vi "Fe Material Properties.vi"(6 "m-nm Fe":dbl, 9 "Fe Thickness":dbl, 10 "Energy (Heat; I^2R)":dbl, 11 "NS Base Area":dbl) -> (1 "Mass Fe":dbl, 2 "Delta Temp Change Fe":dbl, 3 "Fe Specfic Heat Capacity":dbl, 4 "Fe Density":dbl, 5 "Fe Thickness 2":dbl, 7 "Volume Fe":dbl, 8 "mc":dbl)   [LabVIEW 2020]
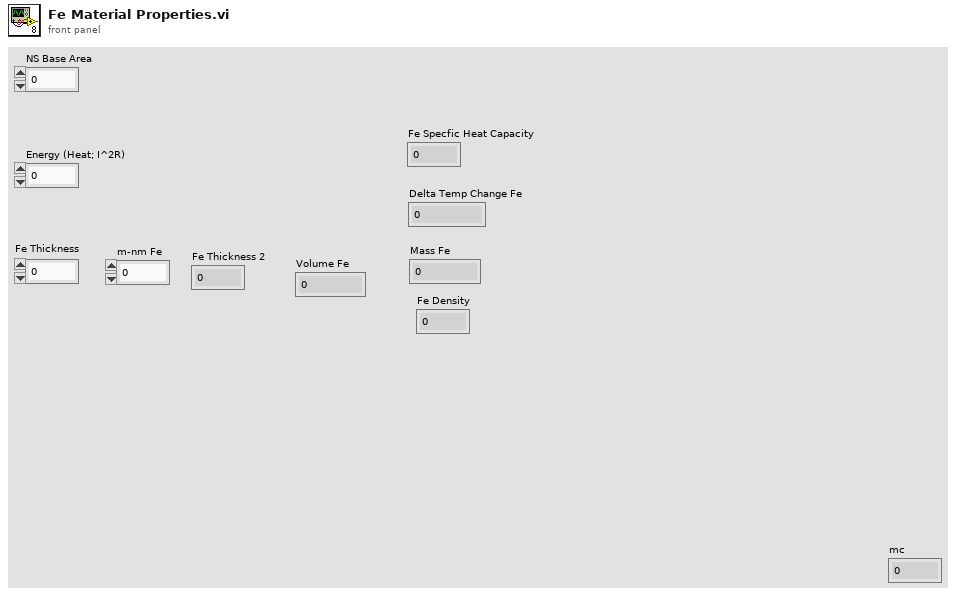
[diagram p1: front panel]
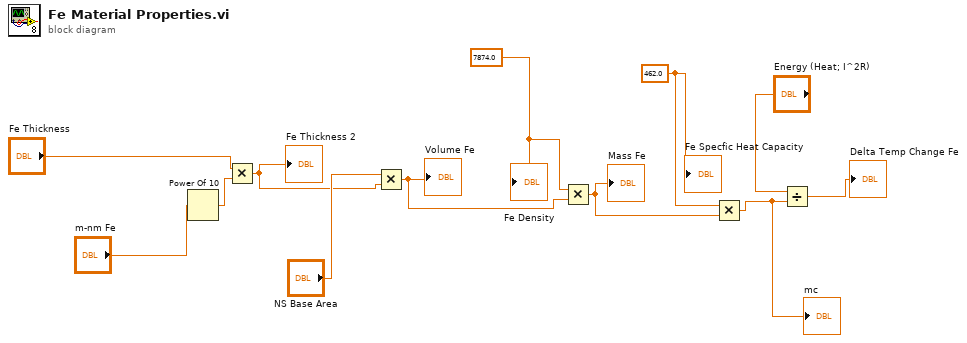
[diagram p0: block diagram]
diagram:
  w12 = 462.0 ("Silicon Specfic Heat Capacity 6")
  w6 = 7874.0 ("Silicon Density 6")
  n1 = Power Of 10(x="m-nm Fe") -> (10^x=w2:dbl)
  n2 = Multiply(x="Fe Thickness", y=w2) -> (x*y=w5:dbl)
  "Fe Thickness 2" <- w5
  n3 = Multiply(x="NS Base Area", y=w5) -> (x*y=w7:dbl)
  "Volume Fe" <- w7
  n4 = Multiply(x=w6, y=w7) -> (x*y=w11:dbl)
  "Mass Fe" <- w11
  n5 = Multiply(x=w12, y=w11) -> (x*y=w1:dbl)
  "mc" <- w1
  n6 = Divide(x="Energy (Heat; I^2R)", y=w1) -> (x/y=→"Delta Temp Change Fe":dbl)
  "Fe Density" <- w6
  "Fe Specfic Heat Capacity" <- w12
